vi "TP 4.3.vi"() -> ()   [LabVIEW 2014]
panel:
  out "XY Graph 3":cluster{"Y":dbl[], "Y":dbl[]}[](graph)
  in  "N2 Muestras":dbl=200.0
  in  "stop":bool
  in  "Amplitud":dbl=1.0
  in  "Frecuencia":dbl=1.0
  in  "N1 Muestras":dbl=100.0
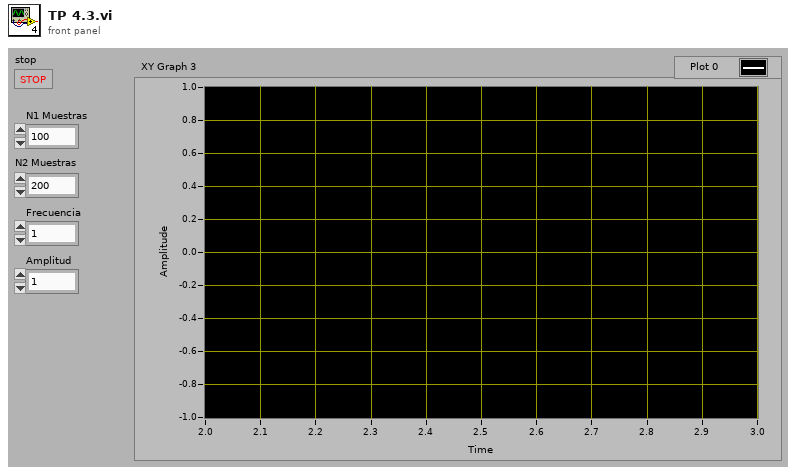
[diagram p1: front panel]
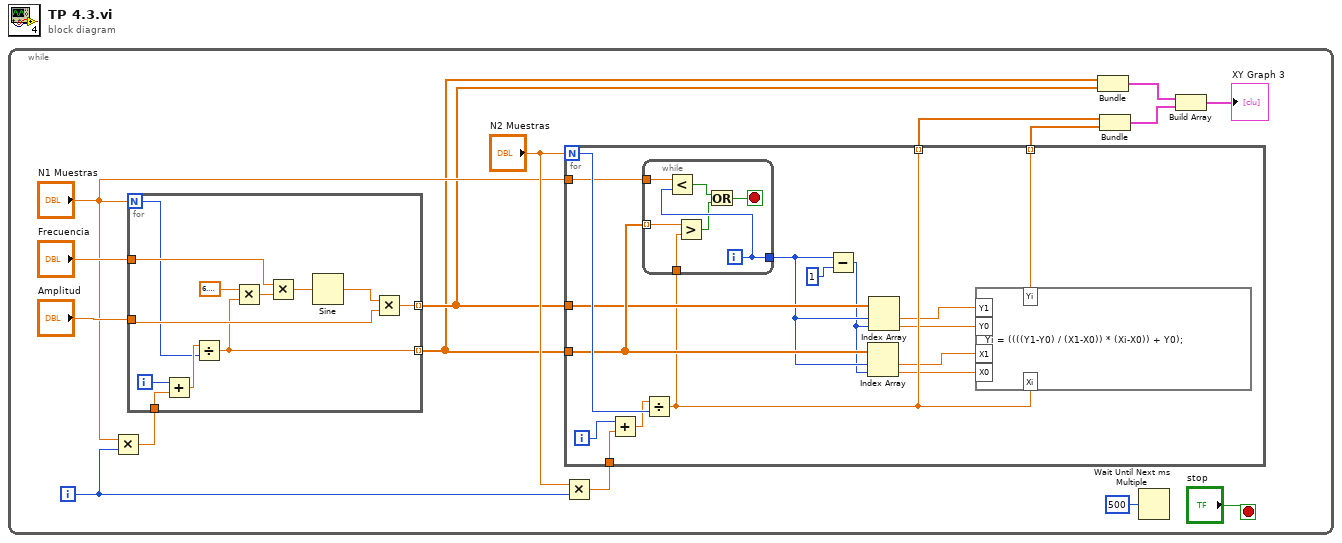
[diagram p0: block diagram]
diagram:
  n1 = while {
    i -> [w11]
    stop <- "stop" stop-if-true
    n2 = Multiply(x="N1 Muestras", y=w11) -> (x*y=w12:dbl)
    n3 = for {
      N: "N1 Muestras" -> [w41]
      tunnel: [w44] -> w7 mode=indexing
      tunnel: w12 -> [w47]
      tunnel: "Frecuencia" -> [w46]
      tunnel: "Amplitud" -> [w45]
      tunnel: [w43] -> w6 mode=indexing
      i -> [w40]
      n4 = Add(x=w40, y=w47) -> (x+y=w42:dbl)
      n5 = Divide(x=w42, y=w41) -> (x/y=w43:dbl)
      n6 = Multiply(x=6.283185307179586, y=w43) -> (x*y=w51:dbl)
      n7 = Multiply(x=w46, y=w51) -> (x*y=w49:dbl)
      n8 = Sine(x=w49) -> (sin(x)=w48:dbl)
      n9 = Multiply(x=w48, y=w45) -> (x*y=w44:dbl)
    }
    n10 = Multiply(x="N2 Muestras", y=w11) -> (x*y=w9:dbl)
    n11 = for {
      N: "N2 Muestras" -> [w32]
      tunnel: w6 -> [w28]
      tunnel: w7 -> [w27]
      tunnel: w9 -> [w30]
      tunnel: [w22] -> w4 mode=indexing
      tunnel: [w21] -> w5 mode=indexing
      tunnel: "N1 Muestras" -> [w23]
      i -> [w29]
      n12 = Add(x=w29, y=w30) -> (x+y=w31:dbl)
      n13 = Divide(x=w31, y=w32) -> (x/y=w22:dbl)
      n14 = while {
        tunnel: w22 -> [w38]
        tunnel: w28 -> [w39] mode=indexing
        tunnel: [w36] -> w26
        tunnel: w23 -> [w37]
        i -> [w36]
        stop <- w35 stop-if-true
        n15 = Less?(x=w37, y=w36) -> (x < y?=w34:bool)
        n16 = Greater?(x=w39, y=w38) -> (0:w33:bool)
        n17 = Or(x=w34, y=w33) -> (x .or. y?=w35:bool)
      }
      n18 = Subtract(x=w26, y=1) -> (x-y=w24:i32)
      n19 = Index Array(array=w28, index #1=w26, index #2=w24) -> (element #1=w18:dbl, element #2=w17:dbl)
      n20 = Index Array(array=w27, index #1=w26, index #2=w24) -> (element #1=w20:dbl, element #2=w19:dbl)
      n21 = formula code="Yi = ((((Y1-Y0) / (X1-X0)) * (Xi-X0)) + Y0);"("X1"=w18, "X0"=w17, "Y1"=w20, "Y0"=w19, "Xi"=w22) -> ("Yi"=w21:dbl)
    }
    n22 = Bundle(w6, w7) -> (w1:cluster{dbl[], dbl[]})  [unwired: 1 in]
    n23 = Bundle(w4, w5) -> (w3:cluster{dbl[], dbl[]})  [unwired: 1 in]
    n24 = Wait Until Next ms Multiple(millisecond multiple=u32 500) -> ()  [unwired: 1 out]
    n25 = Build Array(w1, w3) -> (→"XY Graph 3":cluster{dbl[], dbl[]}[])
  }
